vi "DropVI_SimpleClientSubscriber.vi"() -> ()   [LabVIEW 2023, in "MQTT Client.lvlib"]
uses:
  MQTT Client.lvlib
  Client class/Client.lvclass/Client.ctl
  <vilib>/LabVIEW Open Source Project/MQTT Connection/MQTT_Base/Base Class/MQTT_Base.lvclass/MQTT_Base.ctl
  <vilib>/LabVIEW Open Source Project/Connection/Connection.TCP/Connection.TCP.lvclass
  C:/Program Files (x86)/National Instruments/LabVIEW 2023/vi.lib/LabVIEW Open Source Project/Connection/Connection/Connection.lvclass
  Client class/Client.lvclass
  C:/Program Files (x86)/National Instruments/LabVIEW 2023/vi.lib/LabVIEW Open Source Project/MQTT Connection/MQTT_Base/Base Class/MQTT_Base.lvclass
  <vilib>/LabVIEW Open Source Project/MQTT Control Packets/Control Packets/PUBLISH/PUBLISH.lvclass
  <vilib>/LabVIEW Open Source Project/MQTT Connection/MQTT_Base/Base Class/MQTT_Base.lvclass
  <vilib>/LabVIEW Open Source Project/Connection/Connection/Connection.lvclass
  <vilib>/LabVIEW Open Source Project/Connection/Connection.LocalQueue/Connection.LocalQueue.lvclass
panel:
  out "number":dbl
  out "Payload":u8[](array[numeric]) format="%08b"
  out "loops":i32
  out "Topic":string
  out "last error":errorcluster
  out "Unsuback":bool
  in  "Subscribe":bool
  in  "Connection":bool
  out "Waveform Chart":dbl(graph)
  out "Suback":bool
  in  "Stop Client":bool
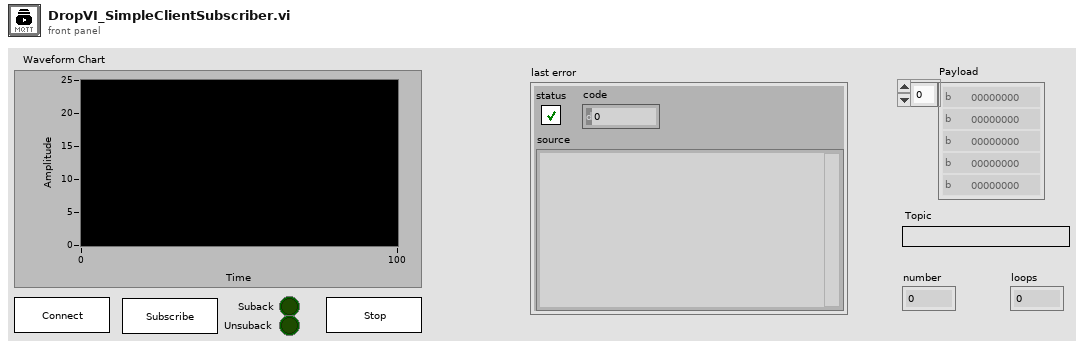
[diagram p1: front panel]
types:
  T1 = typedef "MQTT Client.lvlib/Client.lvclass/Public Events -- cluster.ctl" = cluster{"Connection Status":refnum<user-event>, "Connected":refnum<user-event>, "Application Message":refnum<user-event>}
  T2 = typedef "MQTT Base.lvlib/MQTT_Base.lvclass/Public Events -- cluster.ctl" = cluster{"Stop Event":refnum<user-event>, "Error Event":refnum<user-event>, "Inbound Message":refnum<user-event>}
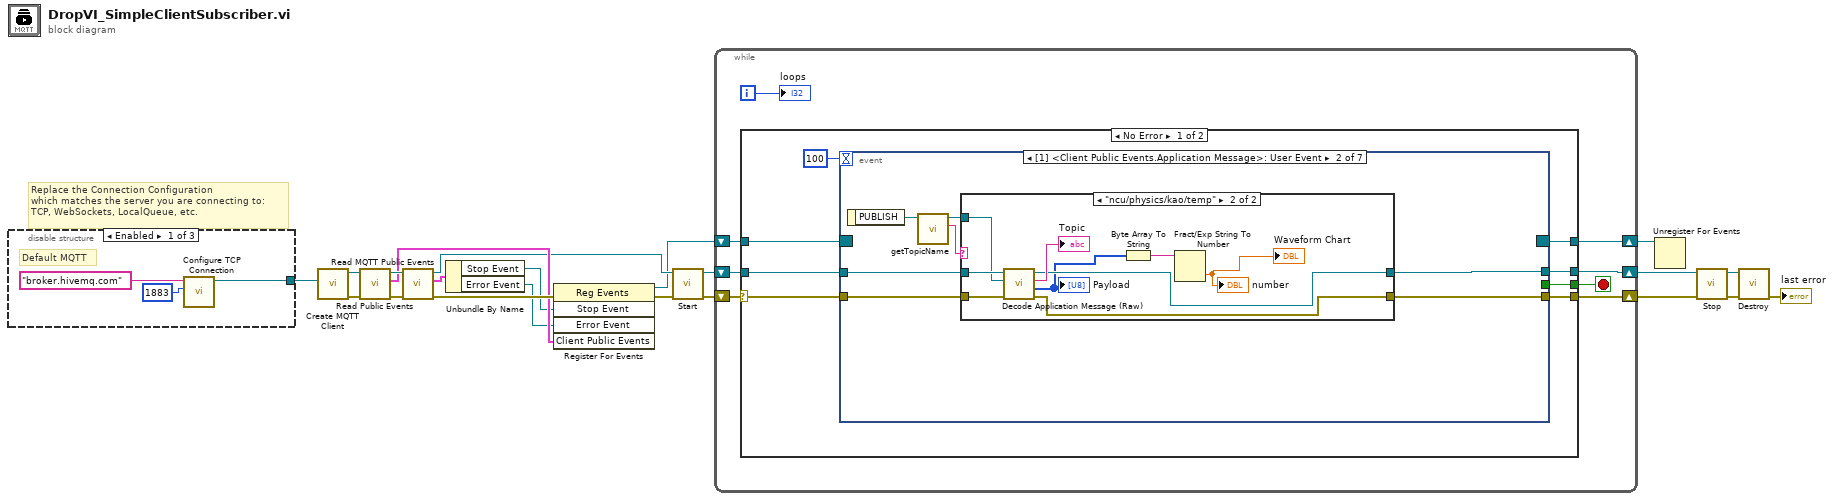
[diagram p0: block diagram]
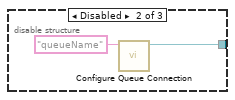
[diagram p2: hidden frame]
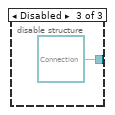
[diagram p3: hidden frame]
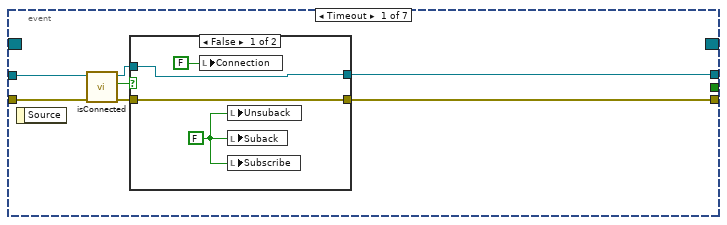
[diagram p4: hidden frame]
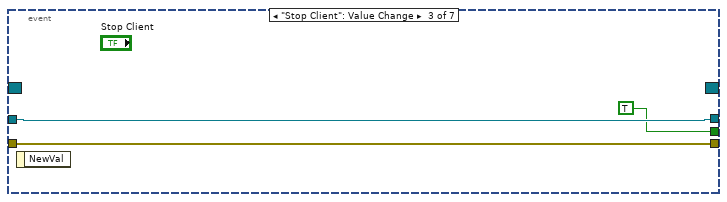
[diagram p7: hidden frame]
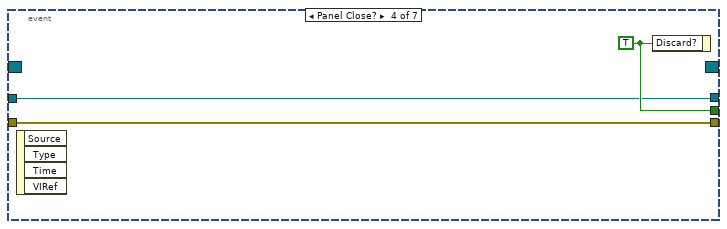
[diagram p8: hidden frame]
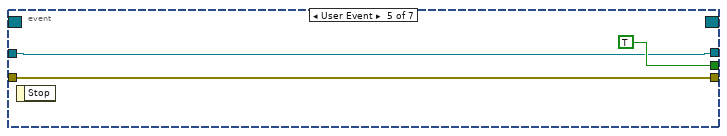
[diagram p9: hidden frame]
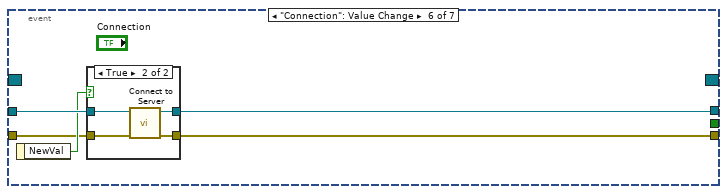
[diagram p10: hidden frame]
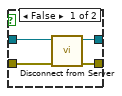
[diagram p11: hidden frame]
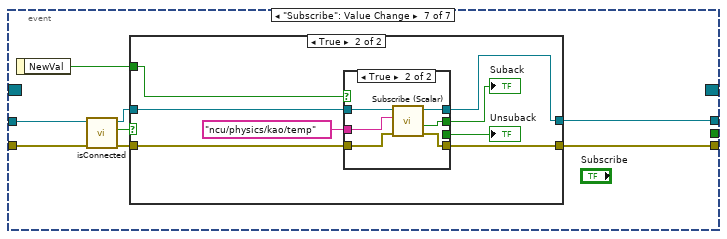
[diagram p12: hidden frame]
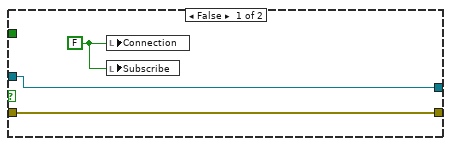
[diagram p13: hidden frame]
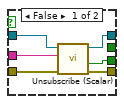
[diagram p14: hidden frame]
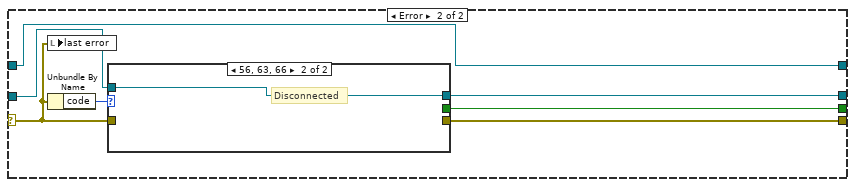
[diagram p15: hidden frame]
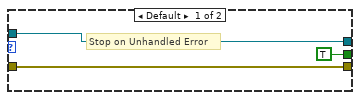
[diagram p16: hidden frame]
diagram:
  # "Replace the Connection Configuration\nwhich matches the server you are connecting to:\nTCP, WebSockets, LocalQueue, etc."
  n1 = disable-structure shown="Enabled" {
    disable-tunnel: [w23 w26 refnum<class "Connection.lvclass"> refnum ("Connection Configuration")] -> w1
    frame Enabled {
      # "Default MQTT"
      n2 = call <vilib>:"Configure TCP Connection.vi"("remote port (80)"=u16 1883, "address (localhost)"="broker.hivemq.com") -> ("Connection.TCP"=w23:refnum<class "Connection.TCP.lvclass">)  [unwired: 8 in, 1 out]
    }
    frame Disabled {
      n3 = call <vilib>:"Configure Queue Connection.vi"("Queue Name"="queueName") -> ("Connection.LocalQueue"=w26:refnum<class "Connection.LocalQueue.lvclass">)  [unwired: 9 in, 1 out]
    }
    frame Disabled {
    }
  }
  n4 = call "Create MQTT Client.vi"("Connection Configuration"=w1) -> ("error out"=w19:errorcluster, "Client out"=w21:refnum<class "Client.lvclass">)  [unwired: 9 in]
  n5 = call "Read Public Events.vi"("error in (no error)"=w19, "Client in"=w21) -> ("error out"=w18:errorcluster, "Client Public Events"=w16:T1, "Client out"=w20:refnum<class "Client.lvclass">)  [unwired: 7 in]
  n6 = call <vilib>:"Read MQTT Public Events.vi"("error in (no error)"=w18, "MQTT_Base in"=w20) -> ("error out"=w17:errorcluster, "MQTT Public Events"=w9:T2, "MQTT_Base out"=w14:refnum<class "Client.lvclass">)  [unwired: 7 in]
  n7 = Unbundle By Name(w9) -> ("Stop Event"=w11:refnum<user-event>, "Error Event"=w10:refnum<user-event>)
  n8 = register-events(error in=w17, w11, w10, w16) -> (reference out=w13:refnum<event-registration>, error out=w15:errorcluster)  [unwired: 1 in]
  n9 = call <vilib>:"Start.vi"("error in (no error)"=w15, "MQTT_Base in"=w14) -> ("error out"=w3:errorcluster, "MQTT_Base out"=w4:refnum<class "Client.lvclass">)  [unwired: 7 in, 1 out]
  n10 = while {
    shift-right: [w34] -> w12
    shift-left: w13 -> [w35]
    shift-right: [w31] -> w7
    shift-left: w4 -> [w32]
    shift-right: [w33] -> w5
    shift-left: w3 -> [w29]
    i -> [w28]
    stop <- w30 stop-if-true
    n11 = case shown="No Error" w29 {
      selector: w29 -> [w36 w131]
      tunnel: w35 -> [w43 w134]
      tunnel: [w42 w134] -> w34
      tunnel: [w41 w129] -> w33
      tunnel: w32 -> [w39 w130]
      tunnel: [w38 w133] -> w31
      tunnel: [w37 w128] -> w30
      frame No Error {
        n12 = event shown="[1] <Client Public Events.Application Message>: User Event" {
          selector: w43 -> [_ _ _ _ _ _ _]
          dyn-events: [_ _ _ _ _ _ _] -> w42
          timeout: 100 -> [_ _ _ _ _ _ _]
          tunnel: w36 -> [w46 w60 w76 w78 w83 w84 w102]
          tunnel: [w49 w57 w76 w78 w83 w85 w103] -> w41
          tunnel: [_ _ TRUE w80 TRUE _ _] -> w37
          tunnel: w39 -> [w48 w61 w77 w79 w81 w88 w101]
          tunnel: [w50 w59 w77 w79 w81 w86 w104] -> w38
          event Timeout {
            n13 = event-data() -> ()  [unwired: 1 in, 1 out]
            n14 = call "isConnected.vi"("error in (no error)"=w46, "Client in"=w48) -> ("error out"=w45:errorcluster, "connected"=w44:bool, "Client out"=w47:refnum<class "Client.lvclass">)  [unwired: 7 in]
            n15 = case shown="False" w44 {
              tunnel: [w54 w56] -> w50
              tunnel: [w53 w55] -> w49
              tunnel: w47 -> [w54 w56]
              tunnel: w45 -> [w53 w55]
              frame False {
                w52 = FALSE
                n16 = local write "Connection"(FALSE ("Connection")) -> ()
                n17 = local write "Unsuback"(w52) -> ()
                n18 = local write "Suback"(w52) -> ()
                n19 = local write "Subscribe"(w52) -> ()
              }
              frame True {
              }
            }
          }
          event User Event {
            n20 = event-data() -> ("PUBLISH"=w63:refnum<class "PUBLISH.lvclass">)  [unwired: 1 in]
            n21 = call <vilib>:"getTopicName.vi"("PUBLISH in"=w63) -> ("Topic"=w58:string, "PUBLISH out"=w62:refnum<class "PUBLISH.lvclass">)  [unwired: 8 in, 1 out]
            n22 = case shown="\"ncu/physics/kao/temp\"" w58 {
              tunnel: w62 -> [_ w72]
              tunnel: w61 -> [w65 w74]
              tunnel: w60 -> [w64 w73]
              tunnel: [w65 w69] -> w59
              tunnel: [w64 w71] -> w57
              frame Default {
              }
              frame "ncu/physics/kao/temp" {
                n23 = call "Decode Application Message (Raw).vi"("error in (no error)"=w73, "PUBLISH"=w72, "Client in"=w74) -> ("error out"=w71:errorcluster, "Payload"=w68:u8[], "Topic"=→"Topic":string, "Client out"=w69:refnum<class "Client.lvclass">)  [unwired: 5 in]
                "Payload" <- w68
                n24 = Byte Array To String(unsigned byte array=w68) -> (string=w67:string)
                n25 = Fract/Exp String To Number(string=w67) -> (number=→"Waveform Chart" →"number":dbl)  [unwired: 3 in, 1 out]
              }
            }
          }
          event "Stop Client": Value Change {
            n26 = event-data() -> ()  [unwired: 1 in, 1 out]
          }
          event Panel Close? {
            w80 = TRUE
            n27 = event-data() -> ()  [unwired: 1 in, 4 out]
            n28 = event-data("Discard?"=w80) -> ()  [unwired: 1 in, 1 out]
          }
          event User Event {
            n29 = event-data() -> ()  [unwired: 1 in, 1 out]
          }
          event "Connection": Value Change {
            n30 = event-data() -> ("NewVal"=w87:bool)  [unwired: 1 in]
            n31 = case shown="True" w87 {
              tunnel: w88 -> [w92 w96]
              tunnel: [w91 w93] -> w86
              tunnel: [w90 w94] -> w85
              tunnel: w84 -> [w89 w95]
              frame False {
                n32 = call "Disconnect from Server.vi"("error in (no error)"=w89, "Client in"=w92) -> ("error out"=w90:errorcluster, "Client out"=w91:refnum<class "Client.lvclass">)  [unwired: 7 in, 1 out]
              }
              frame True {
                n33 = call "Connect to Server.vi"("error in (no error)"=w95, "Client in"=w96) -> ("error out"=w94:errorcluster, "Client out"=w93:refnum<class "Client.lvclass">)  [unwired: 6 in, 2 out]
              }
            }
          }
          event "Subscribe": Value Change {
            n34 = event-data() -> ("NewVal"=w97:bool)  [unwired: 1 in]
            n35 = call "isConnected.vi"("error in (no error)"=w102, "Client in"=w101) -> ("error out"=w99:errorcluster, "connected"=w98:bool, "Client out"=w100:refnum<class "Client.lvclass">)  [unwired: 7 in]
            n36 = case shown="True" w98 {
              tunnel: [w107 w115] -> w104
              tunnel: [w106 w114] -> w103
              tunnel: w100 -> [w107 w113]
              tunnel: w99 -> [w106 w112]
              tunnel: w97 -> [_ w110]
              frame False {
                w105 = FALSE ("Connection")
                n37 = local write "Connection"(w105) -> ()
                n38 = local write "Subscribe"(w105) -> ()
              }
              frame True {
                n39 = case shown="True" w110 {
                  tunnel: [w116 w124] -> w115
                  tunnel: [w117 w123] -> w114
                  tunnel: w113 -> [w121 w127]
                  tunnel: w112 -> [w120 w126]
                  tunnel: "ncu/physics/kao/temp" ("Topic Name (empty: Payload name)") -> [w119 w125]
                  tunnel: [_ w122] -> w109
                  tunnel: [w118 _] -> w108
                  frame False {
                    n40 = call "Unsubscribe (Scalar).vi"("error in (no error)"=w120, "Topic Filter"=w119, "Client in"=w121) -> ("error out"=w117:errorcluster, "Ack"=w118:bool, "Client out"=w116:refnum<class "Client.lvclass">)  [unwired: 6 in]
                  }
                  frame True {
                    n41 = call "Subscribe (Scalar).vi"("error in (no error)"=w126, "Topic Filter"=w125, "Client in"=w127) -> ("error out"=w123:errorcluster, "Ack"=w122:bool, "Client out"=w124:refnum<class "Client.lvclass">)  [unwired: 6 in]
                  }
                }
                "Unsuback" <- w108
                "Suback" <- w109
              }
            }
          }
        }
      }
      frame Error {
        n42 = local write "last error"(w131) -> ()
        n43 = Unbundle By Name(w131) -> ("code"=w132:i32)
        n44 = case shown="56, 63, 66" w132 {
          tunnel: w130 -> [w137 w138]
          tunnel: [w137 w138] -> w133
          tunnel: w131 -> [w136 _]
          tunnel: [w136 _] -> w129
          tunnel: [TRUE _] -> w128
          frame Default {
            # "Stop on Unhandled Error"
          }
          frame 56, 63, 66 {
            # "Disconnected"
          }
        }
      }
    }
    "loops" <- w28
  }
  n45 = Unregister For Events(event registration refnum=w12) -> ()  [unwired: 1 in, 1 out]
  n46 = call <vilib>:"Stop.vi"("error in (no error)"=w5, "MQTT_Base in"=w7) -> ("error out"=w6:errorcluster, "MQTT_Base out"=w8:refnum<class "Client.lvclass">)  [unwired: 7 in, 1 out]
  n47 = call <vilib>:"Destroy.vi"("error in (no error)"=w6, "MQTT_Base in"=w8) -> ("error out"=→"last error":errorcluster)  [unwired: 8 in, 1 out]
